vi "2.vi"() -> ()   [LabVIEW 2015]
uses:
  <vilib>/Utility/sysdir.llb/System Directory Type.ctl
panel:
  out "appended path 2":path
  out "appended path":path
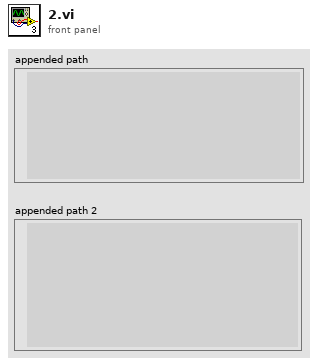
[diagram p1: front panel]
types:
  T1 = typedef "System Directory Type.ctl" = i32
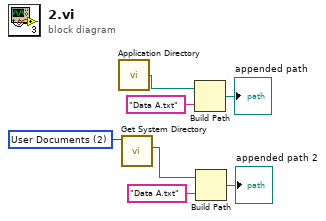
[diagram p0: block diagram]
diagram:
  w1 = T1 2 items=["User Home"=0, "User Desktop"=1, "User Documents"=2, "User Application Data"=3, "User Preferences"=4, "User Temporary"=5, "Public Documents"=6, "Public Application Data"=7, "Public Preferences"=8, "Public Cache"=13, "System Core Libraries"=9, "System Installed Libraries"=10, "Application Files"=11, "Boot Volume Root"=12] ("system directory type")
  n1 = call <vilib>:"Application Directory.vi"() -> ("Application Directory"=w6:path)
  n2 = call <vilib>:"Get System Directory.vi"("system directory type"=w1) -> ("system directory"=w4:path)  [unwired: 10 in]
  n3 = Build Path(base path=w6, name or relative path="Data A.txt") -> (appended path=→"appended path":path)
  n4 = Build Path(base path=w4, name or relative path="Data A.txt") -> (appended path=→"appended path 2":path)
